vi "Update Number of Records Done.vi"(8 "Increment?":bool, 11 "Records Done":u16) -> (3 "Updated Records Done":u16)   [LabVIEW 2012]
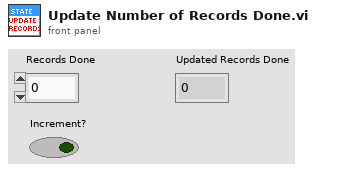
[diagram p1: front panel]
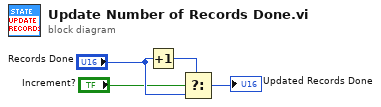
[diagram p0: block diagram]
diagram:
  n1 = Increment(x="Records Done") -> (x+1=w4:u16)
  n2 = Select(t=w4, s="Increment?", f="Records Done") -> (s? t:f=→"Updated Records Done":u16)
